vi "Auton File Loader.vi"   [LabVIEW 2015]
uses:
  Robot Global Data.vi
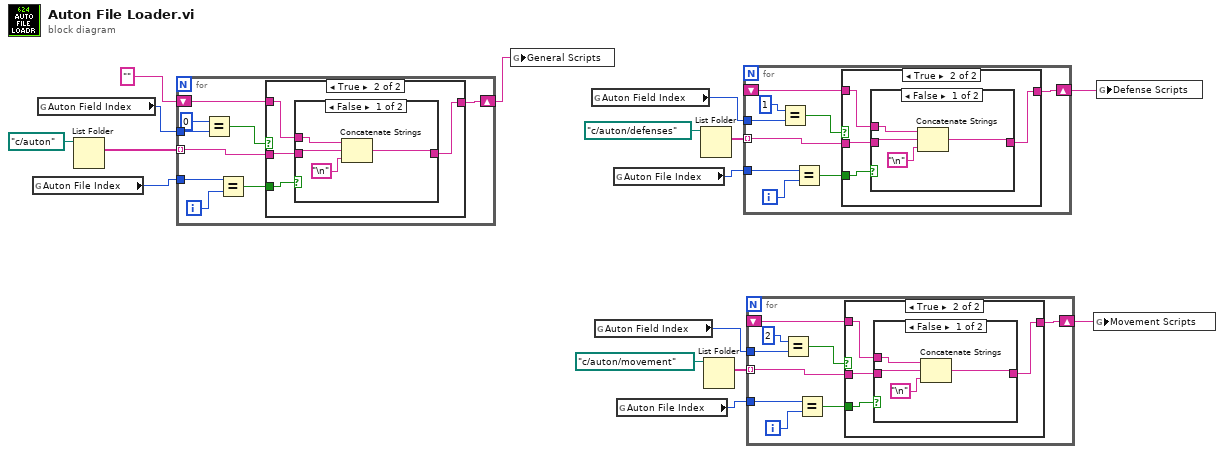
[diagram p0: block diagram]
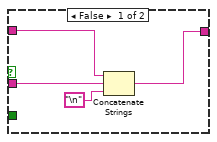
[diagram p2: hidden frame]
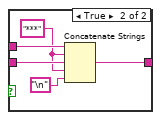
[diagram p3: hidden frame]
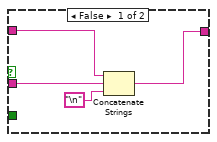
[diagram p4: hidden frame]
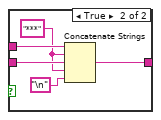
[diagram p5: hidden frame]
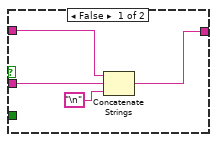
[diagram p6: hidden frame]
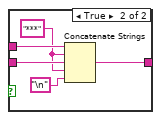
[diagram p7: hidden frame]
diagram:
  n1 = global read "Robot Global Data.vi" "Auton File Index"() -> (w12:i32)
  n2 = global read "Robot Global Data.vi" "Auton Field Index"() -> (w13:i32)
  n3 = List Folder(path=path "c/auton") -> (filenames=w14:string[])  [unwired: 3 in, 3 out]
  n4 = for {
    tunnel: w14 -> [w18] mode=indexing
    tunnel: w13 -> [w25]
    tunnel: w12 -> [w22]
    shift-right: [w17] -> w3
    shift-left: "" -> [w19]
    i -> [w21]
    n5 = Equal?(x=0, y=w25) -> (x = y?=w23:bool)
    n6 = Equal?(x=w22, y=w21) -> (x = y?=w20:bool)
    n7 = case shown="True" w23 {
      tunnel: w20 -> [_ w33]
      tunnel: w19 -> [w29 w32]
      tunnel: w18 -> [w28 w31]
      tunnel: [w26 w30] -> w17
      frame False {
        n8 = Concatenate Strings(w29, w28, "\n") -> (w26:string)
      }
      frame True {
        n9 = case shown="False" w33 {
          tunnel: w32 -> [w37 w42]
          tunnel: w31 -> [w36 w41]
          tunnel: [w34 w38] -> w30
          frame False {
            n10 = Concatenate Strings(w37, w36, "\n") -> (w34:string)
          }
          frame True {
            w40 = "***"
            n11 = Concatenate Strings(w42, w40, w41, w40, "\n") -> (w38:string)
          }
        }
      }
    }
  }
  n12 = global write "Robot Global Data.vi" "General Scripts"(w3) -> ()
  n13 = global read "Robot Global Data.vi" "Auton Field Index"() -> (w9:i32)
  n14 = global read "Robot Global Data.vi" "Auton Field Index"() -> (w6:i32)
  n15 = global read "Robot Global Data.vi" "Auton File Index"() -> (w8:i32)
  n16 = global read "Robot Global Data.vi" "Auton File Index"() -> (w7:i32)
  n17 = List Folder(path=path "c/auton/defenses") -> (filenames=w10:string[])  [unwired: 3 in, 3 out]
  n18 = List Folder(path=path "c/auton/movement") -> (filenames=w5:string[])  [unwired: 3 in, 3 out]
  n19 = for {
    tunnel: w10 -> [w46] mode=indexing
    shift-right: [w45] -> w2
    shift-left: _ -> [w47]
    tunnel: w9 -> [w44]
    tunnel: w8 -> [w43]
    i -> [w49]
    n20 = Equal?(x=1, y=w44) -> (x = y?=w50:bool)
    n21 = Equal?(x=w43, y=w49) -> (x = y?=w48:bool)
    n22 = case shown="True" w50 {
      tunnel: w48 -> [_ w59]
      tunnel: w47 -> [w55 w58]
      tunnel: w46 -> [w54 w57]
      tunnel: [w52 w56] -> w45
      frame False {
        n23 = Concatenate Strings(w55, w54, "\n") -> (w52:string)
      }
      frame True {
        n24 = case shown="False" w59 {
          tunnel: w58 -> [w63 w68]
          tunnel: w57 -> [w62 w67]
          tunnel: [w60 w64] -> w56
          frame False {
            n25 = Concatenate Strings(w63, w62, "\n") -> (w60:string)
          }
          frame True {
            w66 = "***"
            n26 = Concatenate Strings(w68, w66, w67, w66, "\n") -> (w64:string)
          }
        }
      }
    }
  }
  n27 = for {
    tunnel: w5 -> [w72] mode=indexing
    shift-right: [w71] -> w1
    shift-left: _ -> [w73]
    tunnel: w6 -> [w70]
    tunnel: w7 -> [w69]
    i -> [w75]
    n28 = Equal?(x=2, y=w70) -> (x = y?=w76:bool)
    n29 = Equal?(x=w69, y=w75) -> (x = y?=w74:bool)
    n30 = case shown="True" w76 {
      tunnel: w74 -> [_ w85]
      tunnel: w73 -> [w81 w84]
      tunnel: w72 -> [w80 w83]
      tunnel: [w78 w82] -> w71
      frame False {
        n31 = Concatenate Strings(w81, w80, "\n") -> (w78:string)
      }
      frame True {
        n32 = case shown="False" w85 {
          tunnel: w84 -> [w89 w94]
          tunnel: w83 -> [w88 w93]
          tunnel: [w86 w90] -> w82
          frame False {
            n33 = Concatenate Strings(w89, w88, "\n") -> (w86:string)
          }
          frame True {
            w92 = "***"
            n34 = Concatenate Strings(w94, w92, w93, w92, "\n") -> (w90:string)
          }
        }
      }
    }
  }
  n35 = global write "Robot Global Data.vi" "Movement Scripts"(w1) -> ()
  n36 = global write "Robot Global Data.vi" "Defense Scripts"(w2) -> ()
